vi "Robot Global Data.vi"() -> ()   [LabVIEW 2011]
doc: "This global VI can contain as many global variables as you need. Place a control on the panel, give it a good name. To read or write to it from a VI, drag the icon to the diagram of that VI. You can also drag from the project. Click on the node to change which global you access. You shouldn't have multiple locations writing to a global or it will cause a race-condition."
uses:
  <vilib>/Rock Robotics/WPI/Camera/WPI_CameraImageSize.ctl
  <vilib>/Rock Robotics/WPI/DriverStation/WPI_DriverStationRobotMode.ctl
panel:
  in  "Axis":T1 {"J3 Throttle" scale=0.0..10.0; "J3 Y Axis" scale=0.0..10.0; "J2 Y Axis" scale=0.0..10.0; "J1 Y Axis" scale=0.0..10.0}
  out "Set Toggle Speed":dbl
  out "Set Wheel Speed":dbl
  out "Teleop Enabled":T2[](array[typedef])=[enum."Teleop Disabled", enum."Autonomous Disabled", enum."Teleop Enabled", enum."Autonomous Enabled"]
  out "Bottom Wheel Speed":dbl
  out "Top Wheel Speed":dbl
  out "Distance Global":dbl
  in  "Manipulator Buttons":T3
  out "Target Info":T4(array[cluster])
  in  "LED toggle rate (ms)":u32=20
  in  "image size":T5=enum."320x240"
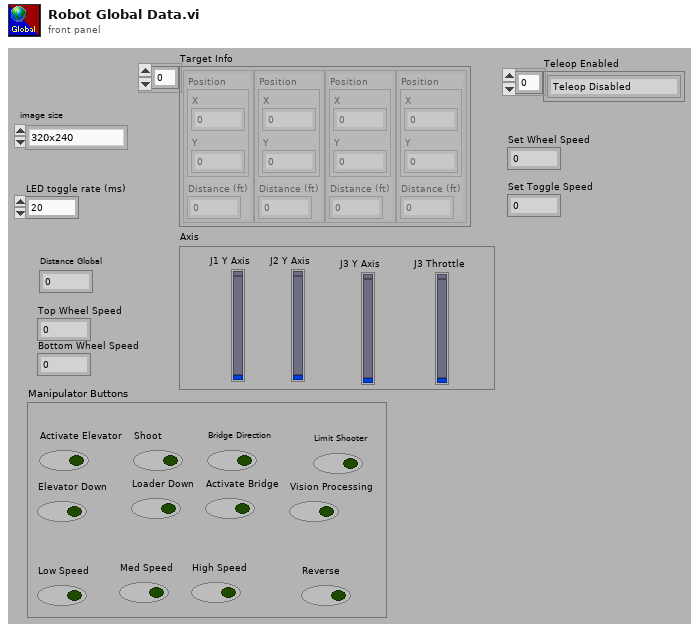
[diagram p1: front panel]
types:
  T1 = cluster{"J1 Y Axis":dbl, "J2 Y Axis":dbl, "J3 Y Axis":dbl, "J3 Throttle":dbl}
  T2 = typedef "WPI_DriverStationRobotMode.ctl" = enum16{"Autonomous Disabled", "Autonomous Enabled", "Teleop Disabled", "Teleop Enabled", "Timeout", "Finish"}
  T3 = cluster{"Activate Elevator":bool, "Shoot":bool, "Bridge Direction":bool, "Low Speed":bool, "Med Speed":bool, "High Speed":bool, "Loader Down":bool, "Activate Bridge":bool, "Limit Shooter":bool, "Elevator Down":bool, "Reverse":bool, "Vision Processing":bool}
  T4 = cluster{"Position":cluster{"X":dbl, "Y":dbl}, "Distance (ft)":dbl}[]
  T5 = typedef "WPI_CameraImageSize.ctl" = enum16{"640x480", "320x240", "160x120"}
diagram:
